vi "Send Position Command.vi"(6 "Polarization":u16(ring) items=["Vertical", "Horizontal"], 8 "error in (no error)":errorcluster, 9 "TR Module/Raster num":i32, 10 "Moves":T1[](array[typedef]), 11 "MotionComm in":refnum<class "MotionComm.lvclass">) -> (0 "error out":errorcluster, 3 "MotionComm out":refnum<class "MotionComm.lvclass">)   [LabVIEW 2018, in "MotionComm.lvclass"]
doc: "Send a command to the VXM thread,\nthen wait for an ack back on the VXM Ack que"
uses:
  MotionComm.lvclass
  APARMainSubvis/VXM Public API/singleAxisMoveDef.ctl
  APARMainSubvis/VXM Public API/mmWaveAxis.ctl
  MotionComm.lvclass/MotionComm.ctl
  Support/MessageQue/MessageQue.lvlib
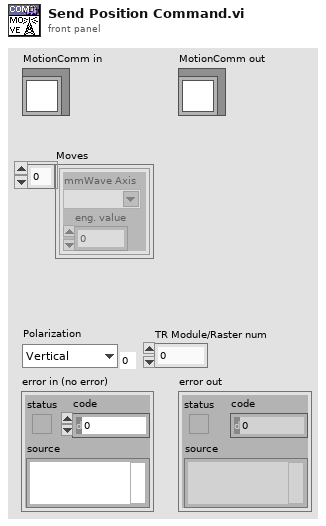
[diagram p1: front panel]
types:
  T1 = typedef "singleAxisMoveDef.ctl" = cluster{"mmWave Axis":T2, "eng. value":dbl}
  T2 = typedef "mmWaveAxis.ctl" = string
  T3 = cluster{"Move Type":string, "Positions":T1[], "Position (Antenna or Raster)":i32, "Polarization":u16}
  T4 = typedef "MessageQue.lvlib/MessageQue.ctl" = refnum<queue>
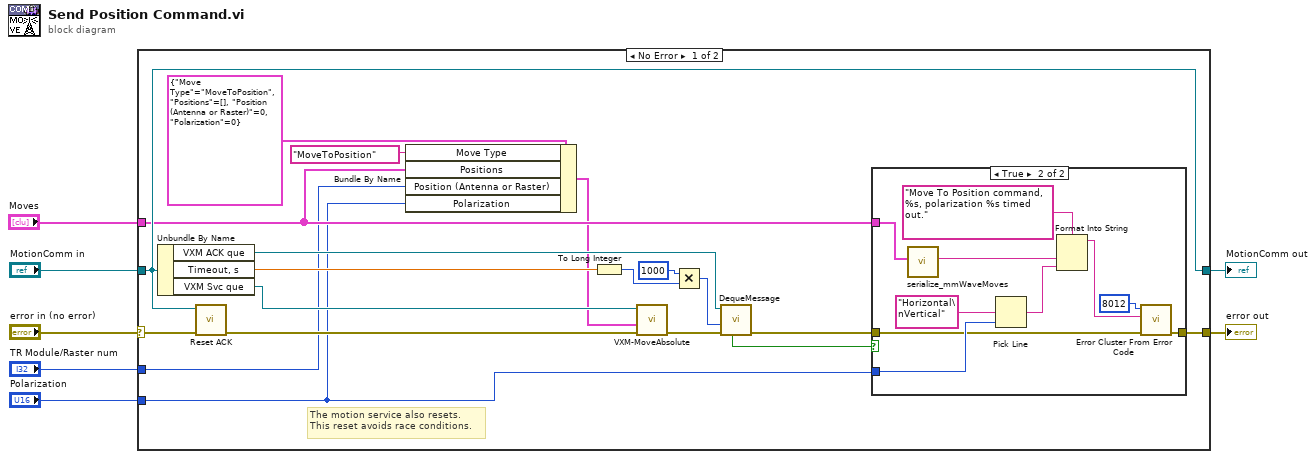
[diagram p0: block diagram]
diagram:
  n1 = case shown="No Error" "error in (no error)" {
    selector: "error in (no error)" -> [w18 w39]
    tunnel: [w19 w39] -> w6
    tunnel: [w17 w38] -> w4
    tunnel: "MotionComm in" -> [w17 w38]
    tunnel: "Polarization" -> [w10 _]
    tunnel: "TR Module/Raster num" -> [w9 _]
    tunnel: "Moves" -> [w11 _]
    frame No Error {
      # "The motion service also resets.\nThis reset avoids race conditions."
      n2 = Unbundle By Name(w17) -> ("VXM ACK que"=w22:T4, "Timeout, s"=w23:dbl, "VXM Svc que"=w16:T4)
      n3 = call "Reset ACK.vi"("error in (no error)"=w18, "MotionComm in"=w17) -> ("error out"=w14:errorcluster)  [unwired: 8 in, 1 out]
      n4 = Bundle By Name(cluster=T3 {"Move Type"="MoveToPosition", "Positions"=[], "Position (Antenna or Raster)"=0, "Polarization"=0} ("Move-Abs"), "Move Type"="MoveToPosition", "Positions"=w11, "Position (Antenna or Raster)"=w9, "Polarization"=w10) -> (w8:T3)
      n5 = To Long Integer(number=w23) -> (32bit integer=w25:i32)
      n6 = call "VXM-MoveAbsolute.vi"("error in (no error)"=w14, "Move-Abs"=w8, "Message que"=w16) -> ("error out"=w15:errorcluster)  [unwired: 8 in]
      n7 = Multiply(x=1000 ("timeout in ms (-1)"), y=w25) -> (x*y=w24:i32)
      n8 = call "DequeMessage.vi"("error in"=w15, "timeout in ms (-1)"=w24, "Message que"=w22) -> ("error out"=w20:errorcluster, "timed out?"=w21:bool)  [unwired: 3 in, 4 out]
      n9 = case shown="True" w21 {
        tunnel: w10 -> [_ w34]
        tunnel: w11 -> [_ w30]
        tunnel: w20 -> [w27 w32]
        tunnel: [w27 w31] -> w19
        frame False {
        }
        frame True {
          n10 = call "serialize_mmWaveMoves.vi"("Moves"=w30) -> ("Moves string"=w29:string)  [unwired: 10 in]
          n11 = Pick Line(multi-line string="Horizontal\nVertical" ("format string"), line index=w34) -> (output string=w28:string)  [unwired: 1 in]
          n12 = Format Into String(format string="Move To Position command, %s, polarization %s timed out.", w29, w28) -> (resulting string=w33:string)  [unwired: 2 in, 1 out]
          n13 = call <vilib>:"Error Cluster From Error Code.vi"("error in (no error)"=w32, "error message (\"\")"=w33, "error code (0)"=8012) -> ("error out"=w31:errorcluster)  [unwired: 6 in]
        }
      }
    }
    frame Error {
    }
  }
  "error out" <- w6
  "MotionComm out" <- w4
